vi "Command Read.vi"() -> (1 "value":i32[](array[numeric]), 3 "command":string[](array[string]))   [LabVIEW 2016]
uses:
  <vilib>/Utility/file.llb/Read Delimited Spreadsheet (string).vi
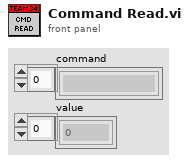
[diagram p1: front panel]
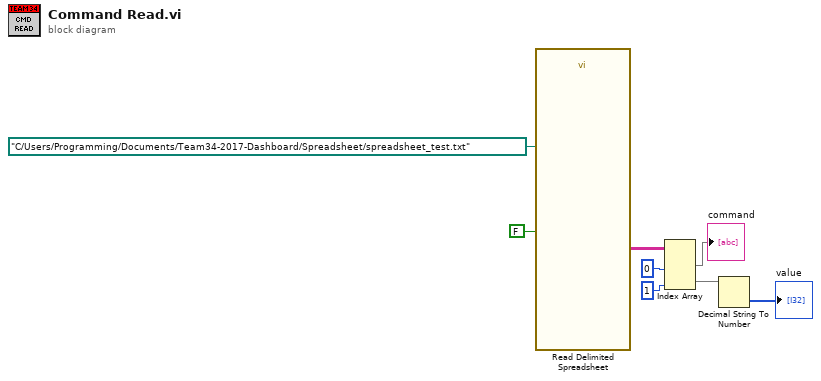
[diagram p0: block diagram]
diagram:
  n1 = call-poly <vilib>:"Read Delimited Spreadsheet.vi"("file path (dialog if empty)"=path "C:/Users/Programming/Documents/Team34-2017-Dashboard/Spreadsheet/spreadsheet_test.txt", "transpose? (F)"=FALSE) -> ("all rows"=w7:string[][])  [unwired: 8 in, 5 out]
  n2 = Index Array(array=w7, index (col) #1=0 ("disabled index (col)"), index (col) #2=1 ("index (col)")) -> (element #1=→"command":string[], element #2=w3:string[])  [unwired: 2 in]
  n3 = Decimal String To Number(string=w3) -> (number=→"value":i32[])  [unwired: 2 in, 1 out]
